vi "AprilTagPoseEstimate_GetAll.vi"(11 "AprilTagPoseEstimate":T5={"AprilTransform3d_1"={"TRANSLATION3D"={"X"=0.0, "Y"=0.0, "Z"=0.0}, "ROTATION3D"={"Q_quaternion"={"R"=1.0, "V"=[0.0, 0.0, 0.0]}}, "XF"=FALSE}, "AprilTransform3d_2"={"TRANSLATION3D"={"X"=0.0, "Y"=0.0, "Z"=0.0}, "ROTATION3D"={"Q_quaternion"={"R"=1.0, "V"=[0.0, 0.0, 0.0]}}, "XF"=FALSE}, "Error1"=0.0, "Error2"=0.0} {"AprilTransform3d_2"."TRANSLATION3D"."Z" format="%14.3f"; "AprilTransform3d_2"."TRANSLATION3D"."Y" format="%14.3f"; "AprilTransform3d_2"."TRANSLATION3D"."X" format="%14.3f"; "AprilTransform3d_1"."TRANSLATION3D"."Z" format="%14.3f"; "AprilTransform3d_1"."TRANSLATION3D"."Y" format="%14.3f"; "AprilTransform3d_1"."TRANSLATION3D"."X" format="%14.3f"}) -> (0 "Error2":dbl, 1 "Error1":dbl, 2 "AprilTransform3d_2":T1={"TRANSLATION3D"={"X"=0.0, "Y"=0.0, "Z"=0.0}, "ROTATION3D"={"Q_quaternion"={"R"=1.0, "V"=[0.0, 0.0, 0.0]}}, "XF"=FALSE} {"TRANSLATION3D"."Z" format="%14.3f"; "TRANSLATION3D"."Y" format="%14.3f"; "TRANSLATION3D"."X" format="%14.3f"}, 3 "AprilTransform3d_1":T1={"TRANSLATION3D"={"X"=0.0, "Y"=0.0, "Z"=0.0}, "ROTATION3D"={"Q_quaternion"={"R"=1.0, "V"=[0.0, 0.0, 0.0]}}, "XF"=FALSE} {"TRANSLATION3D"."Z" format="%14.3f"; "TRANSLATION3D"."Y" format="%14.3f"; "TRANSLATION3D"."X" format="%14.3f"})   [LabVIEW 2019, in "Trajectory_Library.lvlib"]
doc: "Get individual data items from the AprilTagPoseEstimate data cluster.\n\nInputs:\n -- AprilTagPoseEstimate -- AprilTagPoseEstimate -- Input data cluster\n\nOutputs:\n -- AprilTransform3d_1 -- Transform3d -- First april tag transform\n -- AprilTransform3d_1 -- Transform3d -- First april tag transform\n -- Error1 -- double -- Object-space error of pose 1\n -- Error2 -- double -- Object-space error of pose 2"
uses:
  Trajectory_Library.lvlib
  TypeDef/AprilTagPoseEstimate.ctl
  TypeDef/TRANSFORM3D.ctl
  TypeDef/TRANSLATION3D.ctl
  TypeDef/ROTATION3D.ctl
  TypeDef/QUATERNION.ctl
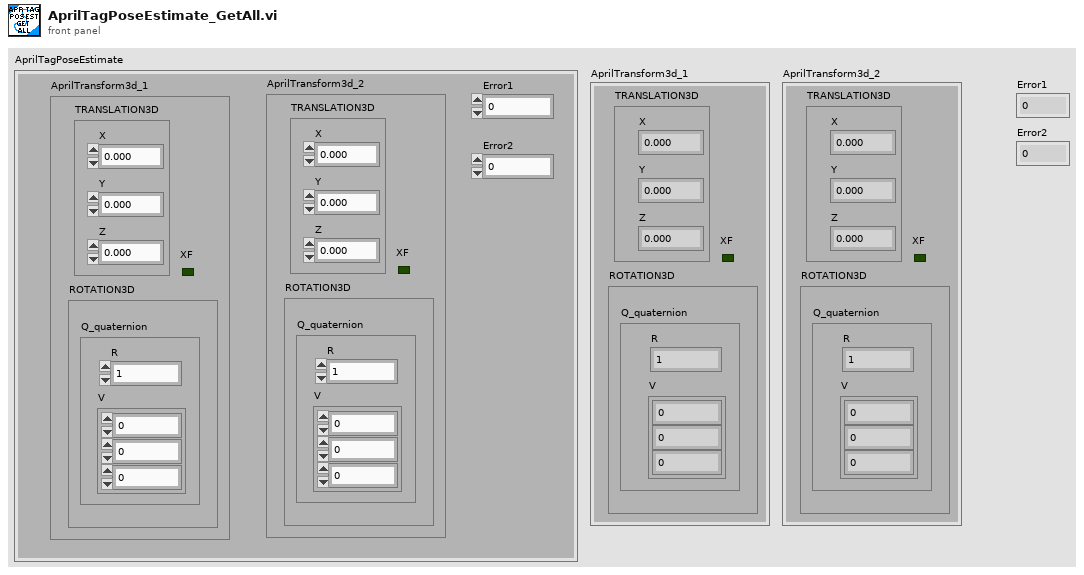
[diagram p1: front panel]
types:
  T1 = typedef "Trajectory_Library.lvlib/TRANSFORM3D.ctl" = cluster{"TRANSLATION3D":T2, "ROTATION3D":T3, "XF":bool}
  T2 = typedef "Trajectory_Library.lvlib/TRANSLATION3D.ctl" = cluster{"X":dbl, "Y":dbl, "Z":dbl}
  T3 = typedef "Trajectory_Library.lvlib/ROTATION3D.ctl" = cluster{"Q_quaternion":T4}
  T4 = typedef "Trajectory_Library.lvlib/QUATERNION.ctl" = cluster{"R":dbl, "V":dbl[]}
  T5 = typedef "Trajectory_Library.lvlib/AprilTagPoseEstimate.ctl" = cluster{"AprilTransform3d_1":T1, "AprilTransform3d_2":T1, "Error1":dbl, "Error2":dbl}
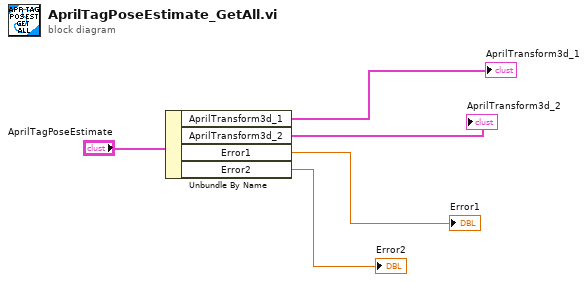
[diagram p0: block diagram]
diagram:
  n1 = Unbundle By Name("AprilTagPoseEstimate") -> ("AprilTransform3d_1"=→"AprilTransform3d_1":T1, "AprilTransform3d_2"=→"AprilTransform3d_2":T1, "Error1"=→"Error1":dbl, "Error2"=→"Error2":dbl)
